vi "Init MICS.vi"(7 "TARGET MICS ID":u32=4358 format="%.0x", 8 "error in (no error)":errorcluster, 11 "VISA Resource Name":refnum<visa-resource-name>) -> (0 "error out":errorcluster, 3 "dup VISA Resource Name":refnum<visa-resource-name>)   [LabVIEW 2010]
uses:
  <vilib>/Instr/_visa.llb/VISA Configure Serial Port (Instr).vi
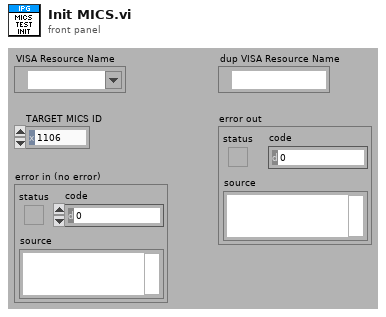
[diagram p1: front panel]
types:
  T1 = cluster{"ConfigFlags":u8, "ImplantID":u32, "CompanyID":u8, "Normal_Comm":cluster{"RF_Channel":u8, "UserData":u8, "TX_Mod":u8, "RX_Mod":u8, "RX_BlockSize":u8, "BlockPerPack":u8, "TX_BlockSize":u8}, "Emerg_Comm":cluster{"RF_Channel":u8, "UserData":u8, "TX_Mod":u8, "RX_Mod":u8, "TX_BlockSize":u8, "BlockPerPack":u8, "RX_BlockSize":u8}, "ImplantRev":u8, "245TX_PowerCal":i8, "245TX_Power":i8, "CCA_RSSI_Thresholds":cluster{"ch0":u16, "ch1":u16, "ch2":u16, "ch3":u16, "ch4":u16, "ch5":u16, "ch6":u16, "ch7":u16, "ch8":u16, "ch9":u16}}
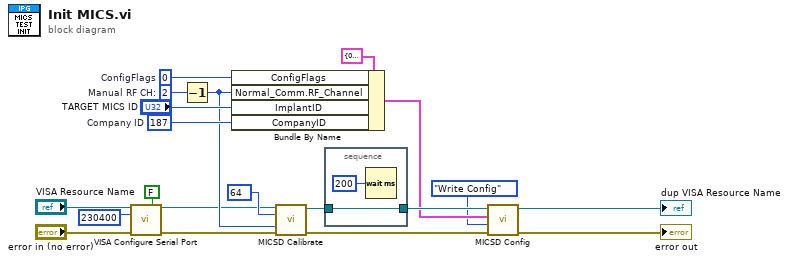
[diagram p0: block diagram]
diagram:
  w18 = u8 0  # ConfigFlags
  w16 = u8 2  # Manual RF CH:
  w15 = u8 187  # Company ID
  n1 = call-poly "VISA Configure Serial Port"("VISA resource name"="VISA Resource Name", "Enable Termination\nChar (T)"=FALSE ("Enable Termination\nChar (T)"), "baud rate (9600)"=u32 230400, "error in (no error)"="error in (no error)") -> ("VISA resource name out"=w5:refnum<visa-resource-name>, "error out"=w4:errorcluster)  [unwired: 10 in]
  n2 = Decrement(x=w16) -> (x-1=w9:u8)
  n3 = Bundle By Name(cluster=T1 {"ConfigFlags"=0, "ImplantID"=1048576, "CompanyID"=187, "Normal_Comm"={"RF_Channel"=4, "UserData"=0, "TX_Mod"=2, "RX_Mod"=8, "RX_BlockSize"=15, "BlockPerPack"=31, "TX_BlockSize"=15}, "Emerg_Comm"={"RF_Channel"=4, "UserData"=0, "TX_Mod"=2, "RX_Mod"=8, "TX_BlockSize"=15, "BlockPerPack"=31, "RX_BlockSize"=15}, "ImplantRev"=4, "245TX_PowerCal"=0, "245TX_Power"=10, "CCA_RSSI_Thresholds"={"ch0"=2650, "ch1"=2650, "ch2"=2650, "ch3"=2650, "ch4"=2650, "ch5"=2650, "ch6"=2650, "ch7"=2650, "ch8"=2650, "ch9"=2650}} ("Default MICS Config"), "ConfigFlags"=w18, "Normal_Comm.RF_Channel"=w9, "ImplantID"="TARGET MICS ID", "CompanyID"=w15) -> (w7:T1)
  n4 = call "MICSD Calibrate.vi"("VISA Resource Name"=w5, "CalSelect1"=u8 64, "Channel"=w9, "error in (no error)"=w4) -> ("dup VISA Resource Name"=w11:refnum<visa-resource-name>, "error out"=w8:errorcluster)  [unwired: 10 in]
  n5 = stacked-sequence {
    tunnel: w11 -> [w21]
    tunnel: [w21] -> w12
    frame #0 {
      n6 = Wait (ms)(milliseconds to wait=u32 200) -> ()  [unwired: 1 out]
    }
  }
  n7 = call "MICSD Config.vi"("error in (no error)"=w8, "Function"=enum16{"Write Config", "Read Config"}."Write Config", "MICS_Config_In"=w7, "VISA Resource Name"=w12) -> ("error out"=→"error out":errorcluster, "dup VISA Resource Name"=→"dup VISA Resource Name":refnum<visa-resource-name>)  [unwired: 5 in, 1 out]
